vi "acqLive.vi"(7 "DVR":T2, 8 "error in":errorcluster, 9 "Save":bool, 10 "img":refnum<queue>) -> (0 "error out":errorcluster, 1 "save?":bool, 2 "Image Out":T1)   [LabVIEW 2020]
uses:
  _controls/data.ref.ctl
  _controls/data.ctl
  _controls/state.ctl
  _controls/data.vars.ctl
  _controls/flip.ctl
  <vilib>/vision/Image Controls.llb/IMAQ Image.ctl
  camera/camera.lvclass
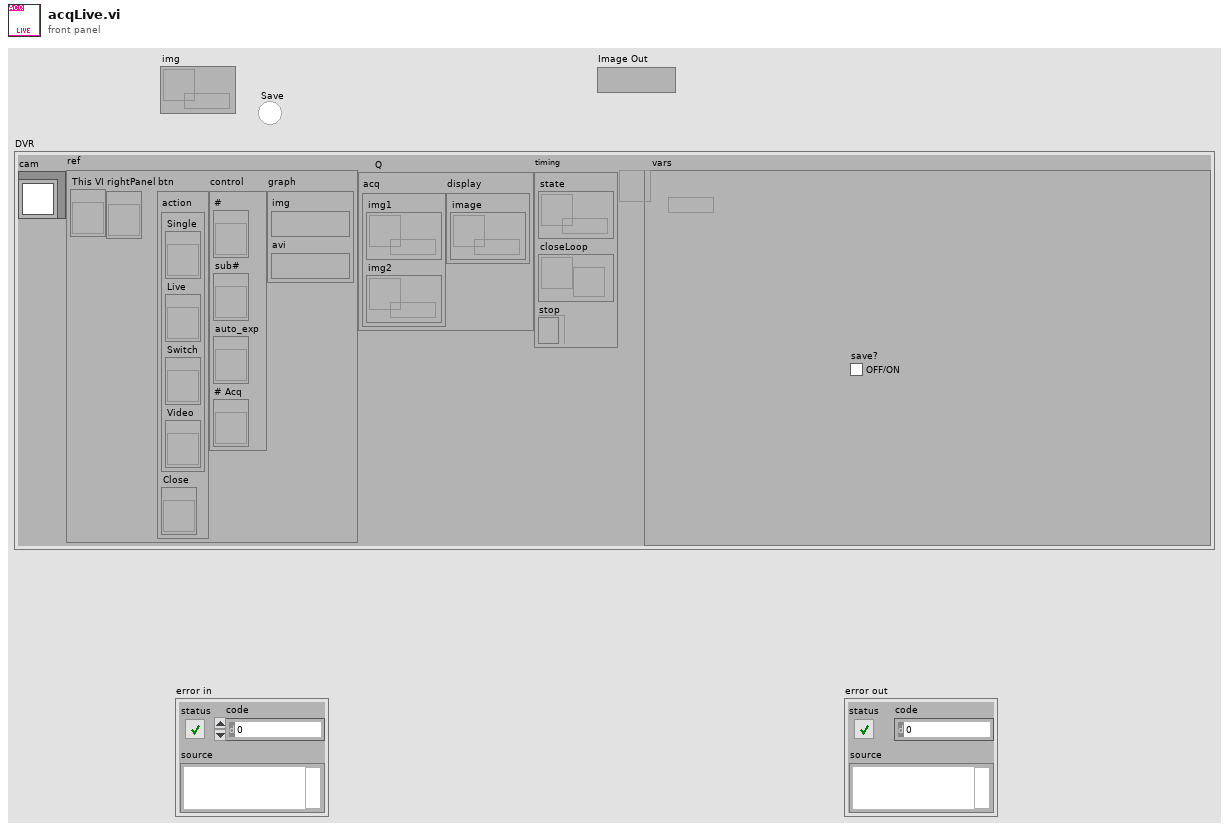
[diagram p1: front panel]
types:
  T1 = typedef "IMAQ Image.ctl" = refnum<image>
  T2 = typedef "data.ctl" = cluster{"cam":refnum<class "camera.lvclass">, "ref":T3, "Q":cluster{"acq":cluster{"img1":refnum<queue>, "img2":refnum<queue>}, "display":cluster{"image":refnum<queue>}}, "timing":cluster{"state":refnum<queue>, "closeLoop":refnum<notifier>, "stop":refnum<k4>}, "vars":refnum<data-value>}
  T3 = typedef "data.ref.ctl" = cluster{"This VI":refnum<vi>, "rightPanel":refnum<vi>, "btn":cluster{"action":cluster{"Single":refnum<vi>, "Live":refnum<vi>, "Switch":refnum<vi>, "Video":refnum<vi>}, "Close":refnum<vi>}, "control":cluster{"#":refnum<vi>, "sub#":refnum<vi>, "auto_exp":refnum<vi>, "# Acq":refnum<vi>}, "graph":cluster{"img":T1, "avi":T1}}
  T4 = typedef "data.vars.ctl" = cluster{"save":cluster{"base_folder":cluster{"Folder":path, "tif":bool, "jpg":bool}, "module":string, "#":u32, "sub#":u8, "save.op":enum16{"Full", "Light"}, "same?":bool, "Shift":enum16{"Single", "Leapfrog"}, "jpg?":bool, "flip":T5}, "acq":cluster{"# Acq":u16, "rotate":bool, "FPS":dbl}, "calib.manual":cluster{"BG":cluster{"Image":u16[][], "enabled?":bool}, "FF":cluster{"Image":u16[][], "enabled?":bool}}}
  T5 = typedef "flip.ctl" = cluster{"x":bool, "y":bool}
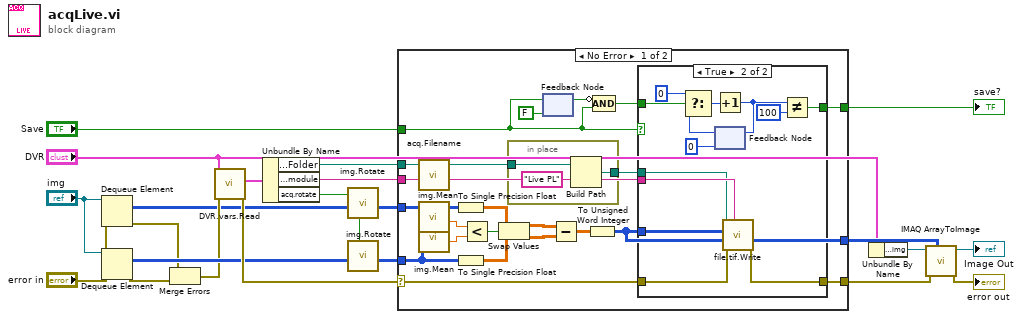
[diagram p0: block diagram]
diagram:
  n1 = Dequeue Element(queue="img", error in (no error)="error in") -> (element=w5:u16[][], error out=w8:errorcluster)  [unwired: 1 in, 2 out]
  n2 = Dequeue Element(queue="img", error in (no error)="error in") -> (element=w9:u16[][], error out=w7:errorcluster)  [unwired: 1 in, 2 out]
  n3 = Merge Errors(w8, w7) -> (w6:errorcluster)
  n4 = call "DVR.vars.Read.vi"("error in"=w6, "DVR.state"="DVR") -> ("error out"=w19:errorcluster, "vars"=w22:T4)  [unwired: 8 in]
  n5 = Unbundle By Name(w22) -> ("save.base_folder.Folder"=w21:path, "save.module"=w20:string, "acq.rotate"=w1:bool)
  n6 = call "img.Rotate.vi"("rotate"=w1, "image in"=w5) -> ("image out"=w4:u16[][])  [unwired: 9 in]
  n7 = call "img.Rotate.vi"("rotate"=w1, "image in"=w9) -> ("image out"=w3:u16[][])  [unwired: 9 in]
  n8 = case shown="No Error" w19 {
    selector: w19 -> [w28 w62]
    tunnel: w21 -> [w39 _]
    tunnel: w20 -> [w43 _]
    tunnel: [w38 w62] -> w15
    tunnel: [w44 _] -> w13
    tunnel: "Save" -> [w42 _]
    tunnel: [w41 _] -> w17
    tunnel: w4 -> [w25 _]
    tunnel: w3 -> [w24 _]
    frame No Error {
      n9 = call "acq.Filename.vi"("module"=w43) -> ("filename"=w40:string)  [unwired: 10 in]
      n10 = call "img.Mean.vi"("IR_img"=w25) -> ("mean"=w26:dbl)  [unwired: 10 in]
      n11 = call "img.Mean.vi"("IR_img"=w24) -> ("mean"=w27:dbl)  [unwired: 10 in]
      n12 = To Single Precision Float(number=w25) -> (single precision float=w23:sgl[][])
      n13 = To Single Precision Float(number=w24) -> (single precision float=w35:sgl[][])
      n14 = Less?(x=w26, y=w27) -> (x < y?=w33:bool)
      n15 = Swap Values(12:w23, 13:w33, 14:w35) -> (1:w32:sgl[][], 3:w34:sgl[][])
      n16 = in-place {
        in-place-border: w39 -> [w61]
        in-place-border: [w59] -> w29
        n17 = Build Path(base path=w61, name or relative path="Live PL") -> (appended path=w59:path)
      }
      n18 = feedback #1(FALSE ("Save")) -> (w37:bool)
      n19 = feedback-in #1(w42) -> ()
      n20 = Subtract(x=w32, y=w34) -> (x-y=w31:sgl[][])
      n21 = To Unsigned Word Integer(number=w31) -> (unsigned 16bit integer=w44:u16[][])
      n22 = Compound Arithmetic op=AND(invert w37, w42) -> (w30:bool)
      n23 = case shown="True" w42 {
        tunnel: w30 -> [_ w52]
        tunnel: w44 -> [_ w51]
        tunnel: [_ w50] -> w41
        tunnel: w28 -> [w45 w49]
        tunnel: [w45 w48] -> w38
        tunnel: w40 -> [_ w47]
        tunnel: w29 -> [_ w46]
        frame False {
        }
        frame True {
          n24 = feedback #2(0) -> (w57:i32)
          n25 = Select(t=0, s=w52, f=w57) -> (s? t:f=w56:i32)
          n26 = Increment(x=w56) -> (x+1=w54:i32)
          n27 = feedback-in #2(w54) -> ()
          n28 = call "file.tif.Write.vi"("name"=w47, "error in"=w49, "u16 pixmap"=w51, "path"=w46) -> ("error out"=w48:errorcluster)  [unwired: 7 in]
          n29 = Not Equal?(x=w54, y=100) -> (x != y?=w50:bool)
        }
      }
    }
    frame Error {
    }
  }
  "save?" <- w17
  n30 = Unbundle By Name("DVR") -> ("ref.graph.img"=w16:T1)
  n31 = call "IMAQ ArrayToImage"("Image Pixels (U16)"=w13, "error in (no error)"=w15, "Image"=w16) -> ("error out"=→"error out":errorcluster, "Image Out"=→"Image Out":T1)  [unwired: 7 in]
